vi "Get Historical Trace.vi"(4 "Archive Database":path=path "\\\\localhost\\c__data", 6 "Logging Database":path=path "\\\\localhost\\c__data", 8 "error in (no error)":errorcluster, 9 "Start Time Stamp":timestamp, 10 "End Time Stamp":timestamp, 11 "Trace Name":refnum<k21>) -> (0 "error out":errorcluster, 3 "Historical Data":T1)   [LabVIEW 2024]
doc: "Gets the historical trace for a given period from the logging database and the archive database. If this trace exists in both databases, the data is merged."
uses:
  Controls/Client/Historical Data.ctl
  <vilib>/lvdsc/historical/Read Trace (Numeric).vi
  <vilib>/lvdsc/NI_DSC.lvlib
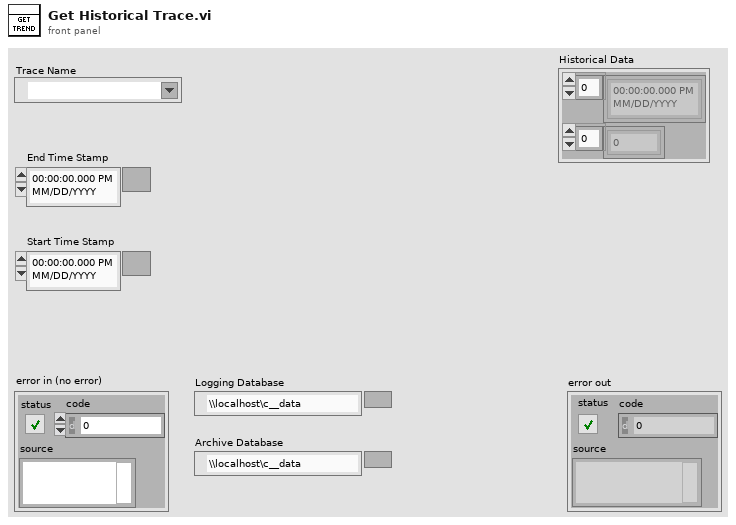
[diagram p1: front panel]
types:
  T1 = typedef "Historical Data.ctl" = cluster{"timestamps":timestamp[], "data":dbl[]}
  T2 = enum16{"Error Case", "From Both Databases", "Only From Archive Database", "Only From Logging Database"}
  T3 = cluster{"start timestamp":timestamp, "stop timestamp (now)":timestamp}
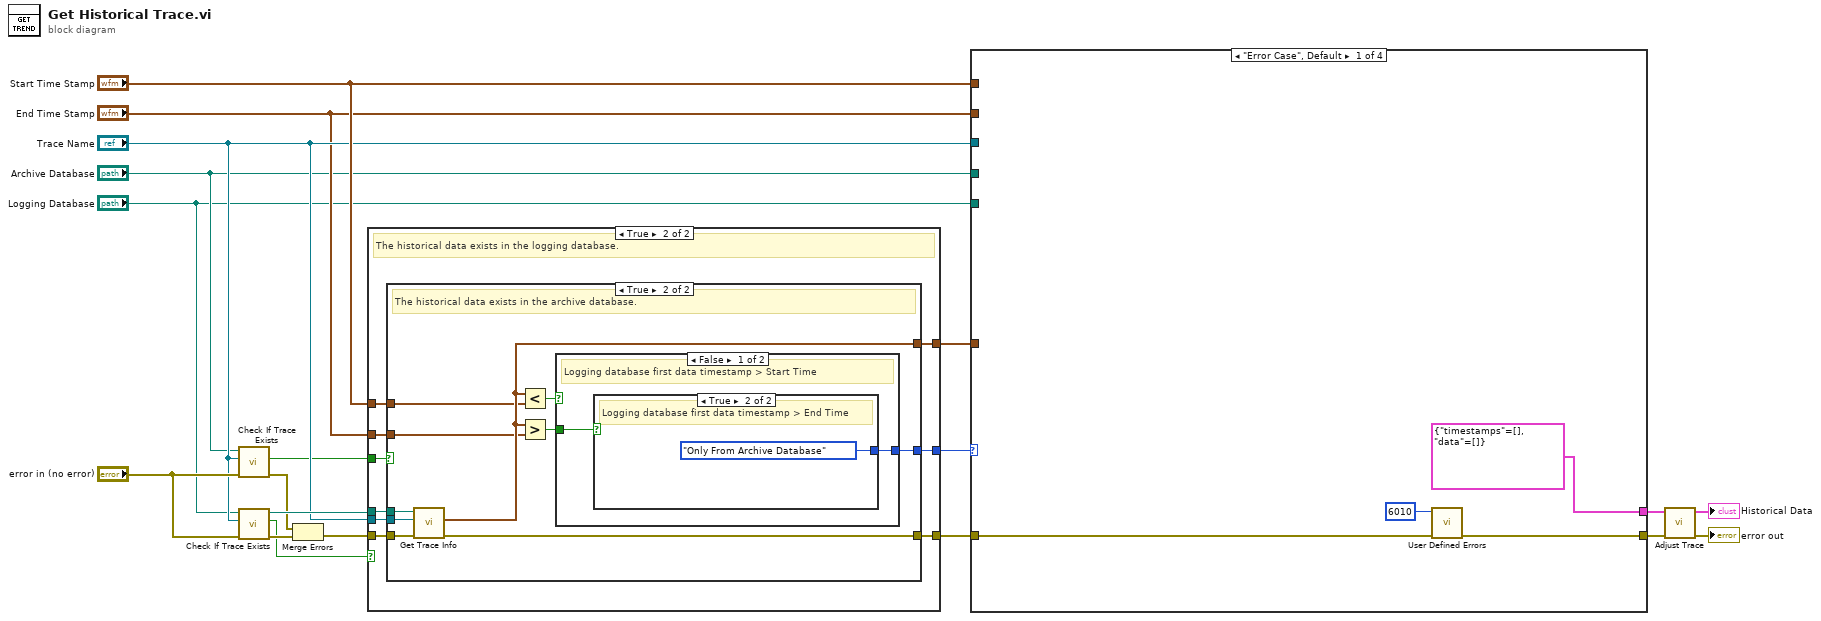
[diagram p0: block diagram]
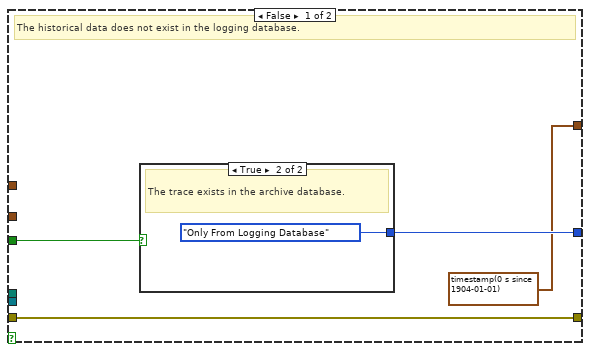
[diagram p2: hidden frame]
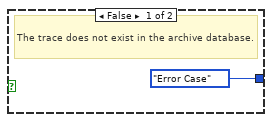
[diagram p3: hidden frame]
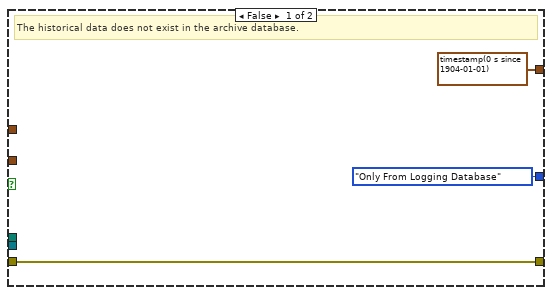
[diagram p4: hidden frame]
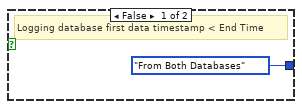
[diagram p5: hidden frame]
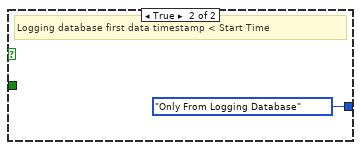
[diagram p6: hidden frame]
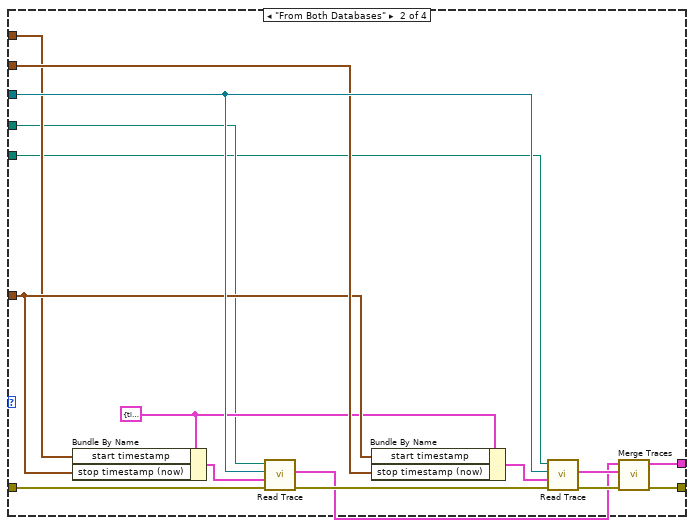
[diagram p7: hidden frame]
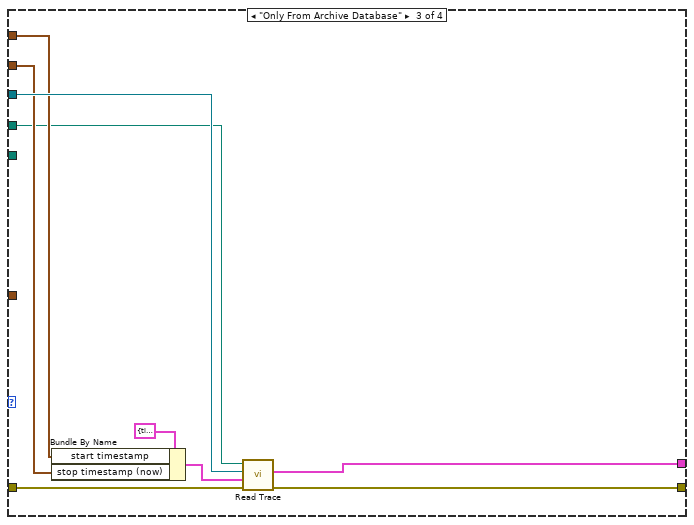
[diagram p8: hidden frame]
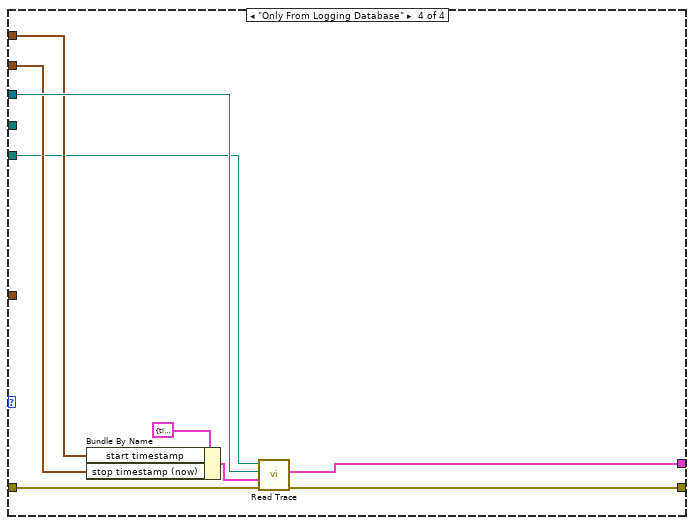
[diagram p9: hidden frame]
diagram:
  n1 = call "Check If Trace Exists.vi"("error in (no error)"="error in (no error)", "Trace Name"="Trace Name", "Database"="Archive Database") -> ("error out"=w16:errorcluster, "Exist?"=w8:bool)  [unwired: 6 in, 1 out]
  n2 = call "Check If Trace Exists.vi"("error in (no error)"="error in (no error)", "Trace Name"="Trace Name", "Database"="Logging Database") -> ("error out"=w15:errorcluster, "Exist?"=w9:bool, "dup Database"=w18:path)  [unwired: 6 in]
  n3 = Merge Errors(w16, w15) -> (w14:errorcluster)
  n4 = case shown="True" w9 {
    tunnel: w18 -> [_ w29]
    tunnel: [timestamp(0 s since 1904-01-01) ("first timestamp") w34] -> w17
    tunnel: w14 -> [w21 w27]
    tunnel: [w23 w33] -> w13
    tunnel: w8 -> [w22 w32]
    tunnel: "Start Time Stamp" -> [_ w31]
    tunnel: "End Time Stamp" -> [_ w30]
    tunnel: "Trace Name" -> [_ w28]
    tunnel: [w21 w26] -> w10
    frame False {
      # "The historical data does not exist in the logging database."
      n5 = case shown="True" w22 {
        tunnel: [T2."Error Case" T2."Only From Logging Database"] -> w23
        frame False {
          # "The trace does not exist in the archive database."
        }
        frame True {
          # "The trace exists in the archive database."
        }
      }
    }
    frame True {
      # "The historical data exists in the logging database."
      n6 = case shown="True" w32 {
        tunnel: [timestamp(0 s since 1904-01-01) ("first timestamp") w47] -> w34
        tunnel: [T2."Only From Logging Database" w38] -> w33
        tunnel: w31 -> [_ w46]
        tunnel: w30 -> [_ w45]
        tunnel: w29 -> [_ w44]
        tunnel: w28 -> [_ w43]
        tunnel: w27 -> [w36 w42]
        tunnel: [w36 w41] -> w26
        frame False {
          # "The historical data does not exist in the archive database."
        }
        frame True {
          # "The historical data exists in the archive database."
          n7 = call <vilib>:"Get Trace Info.vi"("error in (no error)"=w42, "trace name"=w43, "database URL"=w44) -> ("error out"=w41:errorcluster, "first timestamp"=w47:timestamp)  [unwired: 4 in, 3 out]
          n8 = Less?(x=w47, y=w46) -> (x < y?=w40:bool)
          n9 = Greater?(x=w47, y=w45) -> (0:w39:bool)
          n10 = case shown="False" w40 {
            tunnel: w39 -> [w49 _]
            tunnel: [w48 T2."Only From Logging Database"] -> w38
            frame False {
              # "Logging database first data timestamp > Start Time"
              n11 = case shown="True" w49 {
                tunnel: [T2."From Both Databases" T2."Only From Archive Database"] -> w48
                frame False {
                  # "Logging database first data timestamp < End Time"
                }
                frame True {
                  # "Logging database first data timestamp > End Time"
                }
              }
            }
            frame True {
              # "Logging database first data timestamp < Start Time"
            }
          }
        }
      }
    }
  }
  n12 = case shown="\"Error Case\", Default" w13 {
    tunnel: "Trace Name" -> [_ w72 w81 w88]
    tunnel: "End Time Stamp" -> [_ w71 w80 w87]
    tunnel: [cluster{"timestamps":timestamp[], "data":dbl[]} {"timestamps"=[], "data"=[]} ("historical trace") w57 w77 w86] -> w4
    tunnel: [w55 w60 w76 w85] -> w3
    tunnel: w17 -> [_ w70 _ _]
    tunnel: "Start Time Stamp" -> [_ w65 w74 w84]
    tunnel: w10 -> [w53 w62 w75 w83]
    tunnel: "Archive Database" -> [_ w64 w73 _]
    tunnel: "Logging Database" -> [_ w63 _ w82]
    frame "Error Case", Default {
      n13 = call "User Defined Errors.vi"("error in (no error)"=w53, "Error Code (0)"=6010 ("error code (0)")) -> ("error out"=w55:errorcluster)  [unwired: 9 in]
    }
    frame "From Both Databases" {
      w66 = T3 {"start timestamp"=timestamp(0 s since 1904-01-01), "stop timestamp (now)"=timestamp(0 s since 1904-01-01)} ("time interval")
      n14 = Bundle By Name(cluster=w66, "start timestamp"=w65, "stop timestamp (now)"=w70) -> (w69:T3)
      n15 = call-poly <vilib>:"Read Trace.vi"("error in (no error)"=w62, "time interval"=w69, "trace name"=w72, "database URL"=w64) -> ("error out"=w67:errorcluster, "historical trace"=w58:cluster{"timestamps":timestamp[], "data":dbl[]})  [unwired: 4 in, 2 out]
      n16 = Bundle By Name(cluster=w66, "start timestamp"=w70, "stop timestamp (now)"=w71) -> (w68:T3)
      n17 = call-poly <vilib>:"Read Trace.vi"("error in (no error)"=w67, "time interval"=w68, "trace name"=w72, "database URL"=w63) -> ("error out"=w61:errorcluster, "historical trace"=w59:cluster{"timestamps":timestamp[], "data":dbl[]})  [unwired: 4 in, 2 out]
      n18 = call "Merge Traces.vi"("error in (no error)"=w61, "Historical Data from Logging Database"=w59, "Historical Data from Archive Database"=w58) -> ("error out"=w60:errorcluster, "Merged Historical Trace"=w57:T1)  [unwired: 7 in]
    }
    frame "Only From Archive Database" {
      n19 = Bundle By Name(cluster=T3 {"start timestamp"=timestamp(0 s since 1904-01-01), "stop timestamp (now)"=timestamp(0 s since 1904-01-01)} ("time interval"), "start timestamp"=w74, "stop timestamp (now)"=w80) -> (w78:T3)
      n20 = call-poly <vilib>:"Read Trace.vi"("error in (no error)"=w75, "time interval"=w78, "trace name"=w81, "database URL"=w73) -> ("error out"=w76:errorcluster, "historical trace"=w77:cluster{"timestamps":timestamp[], "data":dbl[]})  [unwired: 4 in, 2 out]
    }
    frame "Only From Logging Database" {
      n21 = Bundle By Name(cluster=T3 {"start timestamp"=timestamp(0 s since 1904-01-01), "stop timestamp (now)"=timestamp(0 s since 1904-01-01)} ("time interval"), "start timestamp"=w84, "stop timestamp (now)"=w87) -> (w89:T3)
      n22 = call-poly <vilib>:"Read Trace.vi"("error in (no error)"=w83, "time interval"=w89, "trace name"=w88, "database URL"=w82) -> ("error out"=w85:errorcluster, "historical trace"=w86:cluster{"timestamps":timestamp[], "data":dbl[]})  [unwired: 4 in, 2 out]
    }
  }
  n23 = call "Adjust Trace.vi"("error in (no error)"=w3, "Historical Data In"=w4) -> ("error out"=→"error out":errorcluster, "Historical Data Out"=→"Historical Data":T1)  [unwired: 8 in]
